vi "多通道CAN 回读.vi"(8 "错误输入（无错误）":errorcluster, 9 "枚举":enum16{"CAB500", "CAB1500"}(ring), 10 "Delay Time (s)":dbl=0.2 format="%#_13g") -> (0 "错误输出":errorcluster, 1 "解析电流":dbl, 2 "十次平均":dbl, 3 "报文":string)   [LabVIEW 2021]
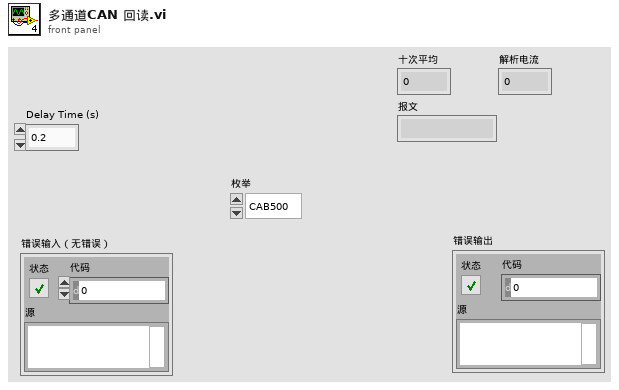
[diagram p1: front panel]
types:
  T1 = cluster{"ID":u32, "MSGTYPE":u8, "LEN":u8, "DATA[0]":u8, "DATA[1]":u8, "DATA[2]":u8, "DATA[3]":u8, "DATA[4]":u8, "DATA[5]":u8, "DATA[6]":u8, "DATA[7]":u8}
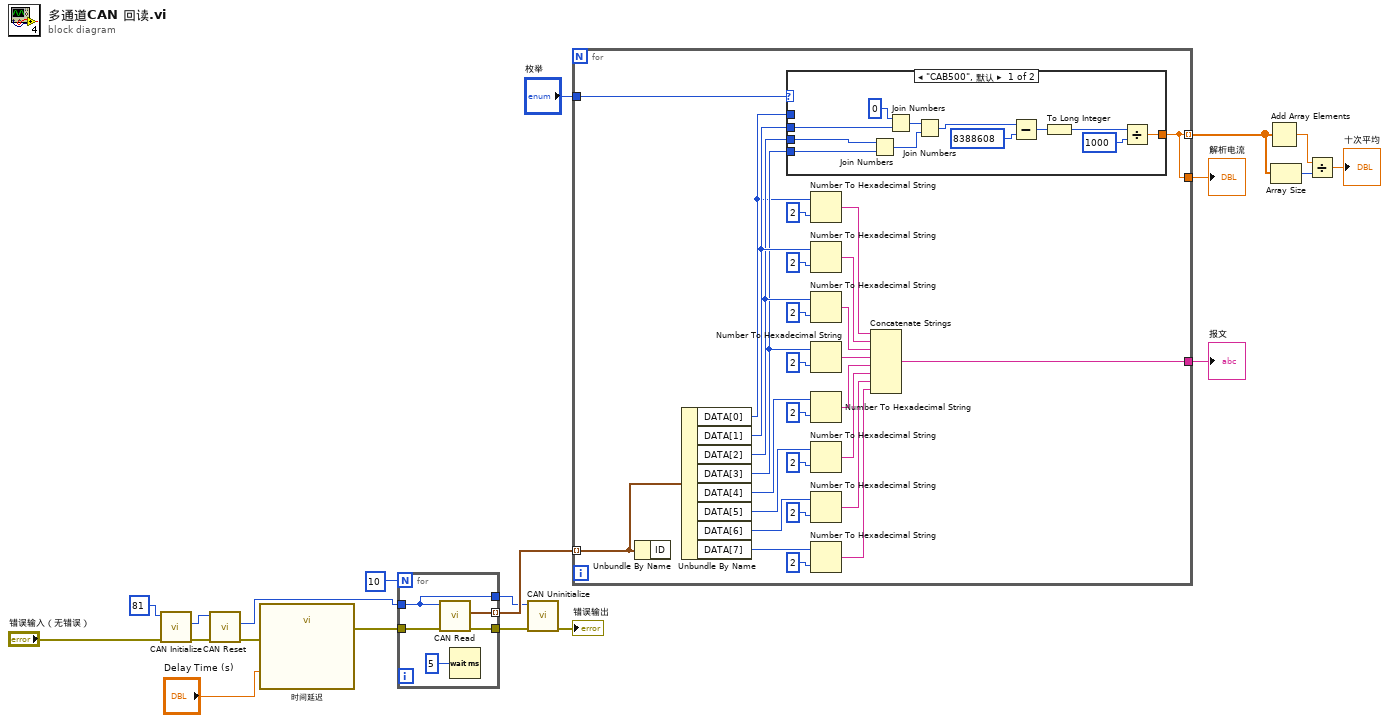
[diagram p0: block diagram]
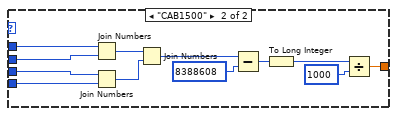
[diagram p2: hidden frame]
diagram:
  n1 = call "CAN Initialize.vi"("错误输入（无错误）"="错误输入（无错误）", "Channel"=u16 81) -> ("错误输出"=w5:errorcluster, "Channel out"=w4:u16)  [unwired: 7 in, 1 out]
  n2 = call "CAN Reset.vi"("错误输入（无错误）"=w5, "Channel in"=w4) -> ("错误输出"=w1:errorcluster, "Channel out"=w3:u16)  [unwired: 7 in, 1 out]
  n3 = call "时间延迟"("error in (no error)"=w1, "Delay Time (s)"="Delay Time (s)") -> ("error out"=w15:errorcluster)  [unwired: 9 in]
  n4 = for {
    N: 10 -> [_]
    tunnel: w3 -> [w23]
    tunnel: [w24] -> w18 mode=indexing
    tunnel: [w23] -> w17
    tunnel: w15 -> [w22]
    tunnel: [w21] -> w16
    n5 = call "CAN Read.vi"("error in (no error)"=w22, "Channel"=w23) -> ("error out"=w21:errorcluster, "MessageBuffer out"=w24:T1)  [unwired: 6 in, 2 out]
    n6 = Wait (ms)(milliseconds to wait=u32 5 ("等待时间（毫秒）")) -> ()  [unwired: 1 out]
  }
  n7 = call "CAN Uninitialize.vi"("error in (no error)"=w16, "Channel"=w17) -> ("error out"=→"错误输出":errorcluster)  [unwired: 8 in, 1 out]
  n8 = for {
    tunnel: w18 -> [w53] mode=indexing
    tunnel: [w52] -> w10
    tunnel: [w26] -> w13 mode=indexing
    tunnel: "枚举" -> [w27]
    tunnel: [w26] -> w8
    n9 = Unbundle By Name(w53) -> ()  [unwired: 1 out]
    n10 = Unbundle By Name(w53) -> ("DATA[0]"=w28:u8, "DATA[1]"=w31:u8, "DATA[2]"=w30:u8, "DATA[3]"=w29:u8, "DATA[4]"=w43:u8, "DATA[5]"=w42:u8, "DATA[6]"=w41:u8, "DATA[7]"=w40:u8)
    n11 = case shown="\"CAB500\", 默认" w27 {
      tunnel: [w57 w77] -> w26
      tunnel: w31 -> [w56 w68]
      tunnel: w30 -> [w55 w67]
      tunnel: w29 -> [w54 w66]
      tunnel: w28 -> [_ w69]
      frame "CAB500", Default {
        n12 = Join Numbers(hi=w55, lo=w54) -> ((hi.lo)=w64:u16)
        n13 = Join Numbers(hi=u8 0, lo=w56) -> ((hi.lo)=w59:u16)
        n14 = Join Numbers(hi=w59, lo=w64) -> ((hi.lo)=w60:u32)
        n15 = Subtract(x=w60, y=u32 8388608) -> (x-y=w63:u32)
        n16 = To Long Integer(number=w63) -> (32bit integer=w62:i32)
        n17 = Divide(x=w62, y=1000) -> (x/y=w57:dbl)
      }
      frame "CAB1500" {
        n18 = Join Numbers(hi=w69, lo=w68) -> ((hi.lo)=w70:u16)
        n19 = Join Numbers(hi=w67, lo=w66) -> ((hi.lo)=w75:u16)
        n20 = Join Numbers(hi=w70, lo=w75) -> ((hi.lo)=w71:u32)
        n21 = Subtract(x=w71, y=u32 8388608) -> (x-y=w74:u32)
        n22 = To Long Integer(number=w74) -> (32bit integer=w73:i32)
        n23 = Divide(x=w73, y=1000) -> (x/y=w77:dbl)
      }
    }
    n24 = Number To Hexadecimal String(1:i16 2 ("宽度(-)"), 2:w28) -> (0:w39:string)
    n25 = Number To Hexadecimal String(1:i16 2 ("宽度(-)"), 2:w31) -> (0:w38:string)
    n26 = Number To Hexadecimal String(1:i16 2 ("宽度(-)"), 2:w30) -> (0:w37:string)
    n27 = Number To Hexadecimal String(1:i16 2 ("宽度(-)"), 2:w29) -> (0:w36:string)
    n28 = Number To Hexadecimal String(1:i16 2 ("宽度(-)"), 2:w43) -> (0:w35:string)
    n29 = Number To Hexadecimal String(1:i16 2 ("宽度(-)"), 2:w42) -> (0:w34:string)
    n30 = Number To Hexadecimal String(1:i16 2 ("宽度(-)"), 2:w41) -> (0:w33:string)
    n31 = Number To Hexadecimal String(1:i16 2 ("宽度(-)"), 2:w40) -> (0:w32:string)
    n32 = Concatenate Strings(w39, w38, w37, w36, w35, w34, w33, w32) -> (w52:string)
  }
  "报文" <- w10
  "解析电流" <- w8
  n33 = Add Array Elements(numeric array=w13) -> (sum=w12:dbl)
  n34 = Array Size(array=w13) -> (size(s)=w11:i32)
  n35 = Divide(x=w12, y=w11) -> (x/y=→"十次平均":dbl)
